vi "autofocus-globals.vi"() -> ()   [LabVIEW 2014]
panel:
  in  "Shutter Camera\nduring calibration?":bool
  out "TIRF - Handle":u32
  in  "Max iterations \nper autofocus":i32=3 min=1
  in  "Number of sensor\nreadings to average":i32=2 min=1 step=1
  in  "Set focus point\nto current z position":bool
  in  "Manual focus\noffset (um)":dbl
  in  "Repeat AF if delta z \ngreater than (um)":dbl=1.0
  in  "Focus direction is X":bool
  in  "Sensor number (1-4)":i8=12 min=1 max=4 step=1
  in  "Warn if power \nless than":dbl=0.0001
  in  "RR calibration curve multi-step\nadd'l settle time (ms)":u16=3000
  in  "RR calibration curve\nsettle time (ms)":u16=5000
  in  "RR calibration curve\nhalf-width  (steps)":u16=15
  in  "RR calibration curve\nstep size (um)":ext=0.150000000000000000005
  in  "Calibration curve":cluster{"z (um)":ext[], "QPD position":dbl[]}
  out "Acquiring from QPD":bool
  in  "Asynchronous autofocus?":bool
  in  "AF every N seconds during Wait; 0 = don't":u16
  in  "AF every Nth cycle, N =":u8=1
  in  "Focus Mode":T1(radio)
  # "Multi-Mode Acquisition"
  # "Autofocus"
  # "Calibration"
  # "General"
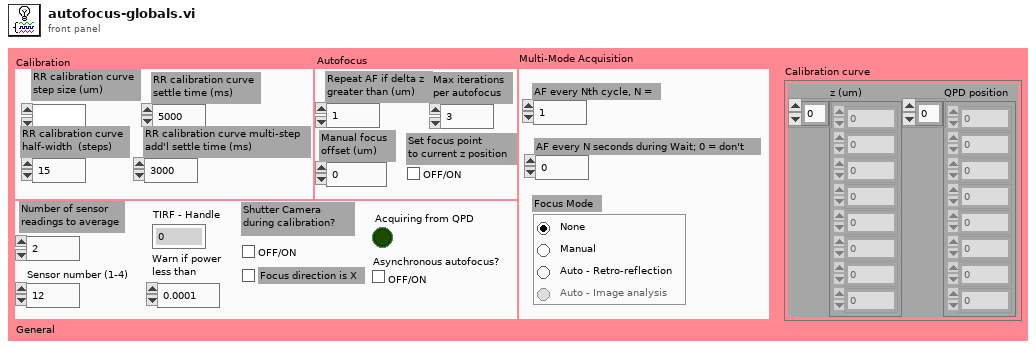
[diagram p1: front panel]
types:
  T1 = enum32{"None", "Manual", "Auto - Image analysis", "Auto - Retro-reflection"}
diagram:
